vi "Index Array Function.vi"() -> ()   [LabVIEW 2012]
panel:
  out "提取的列":i32[](array[numeric])
  out "提取的元素":i32
  out "提取的行":i32[](array[numeric])
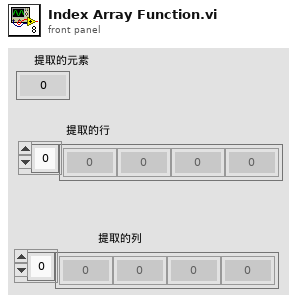
[diagram p1: front panel]
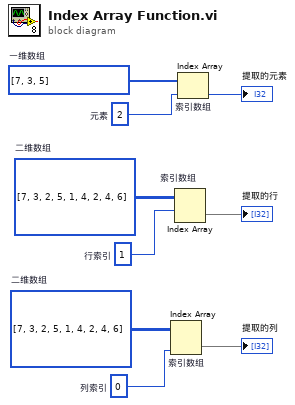
[diagram p0: block diagram]
diagram:
  w1 = 0  # 列索引
  w2 = i32[][] [[7, 3, 2], [5, 1, 4], [2, 4, 6]]  # 二维数组
  w6 = 1  # 行索引
  w7 = i32[][] [[7, 3, 2], [5, 1, 4], [2, 4, 6]]  # 二维数组
  w8 = 2  # 元素
  w9 = i32[] [7, 3, 5]  # 一维数组
  n1 = Index Array "索引数组"(array=w2, index (col)=w1) -> (element=→"提取的列":i32[])  [unwired: 1 in]
  n2 = Index Array "索引数组"(array=w7, index (row)=w6) -> (element=→"提取的行":i32[])  [unwired: 1 in]
  n3 = Index Array "索引数组"(array=w9, index=w8) -> (element=→"提取的元素":i32)
